vi "송신수신01.vi"() -> ()   [LabVIEW 2014]
panel:
  in  "정지":bool
  out "데이터 출력":string
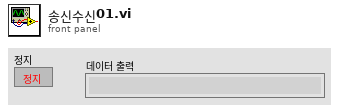
[diagram p1: front panel]
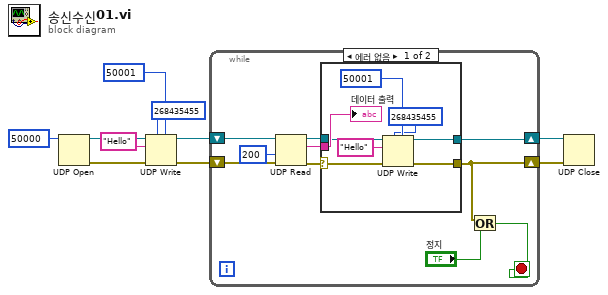
[diagram p0: block diagram]
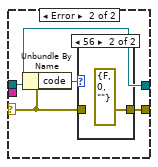
[diagram p2: hidden frame]
diagram:
  n1 = UDP Open(11:u16 50000 ("포트")) -> (port=w3:refnum<k16>, 0:w2:errorcluster)  [unwired: 4 in, 1 out]
  n2 = UDP Write(address=u32 268435455 ("주소"), port or service name=u16 50001 ("포트 또는 서비스 이름"), connection ID=w3, data in="Hello" ("데이터 입력"), 8:w2) -> (error out=w1:errorcluster, 3:w4:refnum<k16>)  [unwired: 1 in]
  n3 = while {
    shift-right: [w11] -> w10
    shift-left: w4 -> [w20]
    shift-right: [w13] -> w9
    shift-left: w1 -> [w19]
    stop <- w17 stop-if-true
    n4 = UDP Read(connection ID=w20, timeout ms (25000)=200 ("타임아웃 ms (25000)"), 8:w19) -> (data out=w18:string, error out=w14:errorcluster, 3:w12:refnum<k16>)  [unwired: 1 in, 2 out]
    n5 = case shown="에러 없음" w14 {
      selector: w14 -> [w24 w30]
      tunnel: w18 -> [w28 _]
      tunnel: [w25 w31] -> w13
      tunnel: w12 -> [w27 w29]
      tunnel: [w26 w29] -> w11
      frame No Error {
        n6 = UDP Write(address=u32 268435455 ("주소"), port or service name=u16 50001 ("포트 또는 서비스 이름"), connection ID=w27, data in="Hello" ("데이터 입력"), 8:w24) -> (error out=w25:errorcluster, 3:w26:refnum<k16>)  [unwired: 1 in]
        "데이터 출력" <- w28
      }
      frame Error {
        n7 = Unbundle By Name(w30) -> ("code"=w32:i32)
        n8 = case shown="56" w32 {
          tunnel: [w33 errorcluster {"status"=FALSE, "code"=0, "source"=""} ("에러 상수")] -> w31
          tunnel: w30 -> [w33 _]
          frame Default {
          }
          frame 56 {
          }
        }
      }
    }
    n9 = Or(x=w13, y="정지") -> (x .or. y?=w17:bool)
  }
  n10 = UDP Close(connection ID=w10, 8:w9) -> ()  [unwired: 2 out]
